vi "Init.vi"(6 "Creator":refnum<user-event>, 8 "Creator Alias":string, 9 "Self":refnum<user-event>, 10 "Self Alias":string) -> (3 "Base Addresses Strategy out":refnum<class "Base Addresses Strategy.lvclass">)   [LabVIEW 2021, in "jettl.lvlib" / "Addresses Strategy.lvlib" / "Base Addresses Strategy.lvclass"]
uses:
  Base Addresses Strategy.lvclass
  Msg Strategy/Msg Strategy.lvclass
  Base Addresses Strategy.lvclass/Base Addresses Strategy.ctl
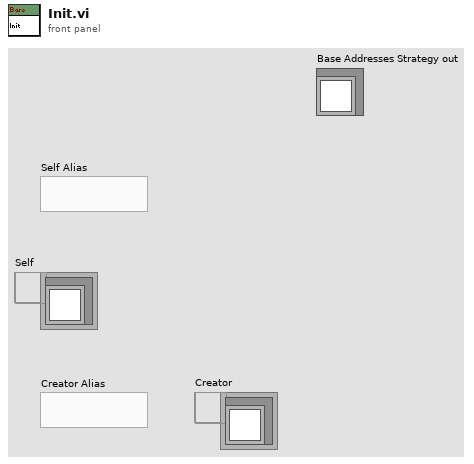
[diagram p1: front panel]
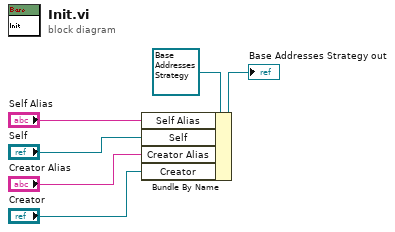
[diagram p0: block diagram]
diagram:
  n1 = Bundle By Name(cluster=refnum<class "Base Addresses Strategy.lvclass"> refnum ("Queue Mailbox out"), "Self Alias"="Self Alias", "Self"="Self", "Creator Alias"="Creator Alias", "Creator"="Creator") -> (→"Base Addresses Strategy out":refnum<class "Base Addresses Strategy.lvclass">)
